vi "TI sbRIO Main (FPGA).vi"() -> ()   [LabVIEW 2019]
uses:
  Type Defs/Controller Names.ctl
  <vilib>/Platform/TimedLoop/XDataNode/timing_clust.ctl
  <vilib>/Platform/TimedLoop/XDataNode/nitl_modes.ctl
  <vilib>/Platform/TimedLoop/XDataNode/wakeup.ctl
  <vilib>/rvi/FXPMathLib/basic elements/FxpIntAccumulator/subVIs/nifxpmath_IntAccumulator_SimConfig.ctl
  <vilib>/rvi/FXPMathLib/FxpSqrt/subVIs/nifxpmath_Sqrt_SimConfig.ctl
  <vilib>/fxp/LVFixedPointOverflowPolicyTypeDef.ctl
  <vilib>/rvi/FXPMathLib/FxpDiv/subVIs/nifxpmath_Div_SimConfig.ctl
  <vilib>/rvi/Emulation/niFpgaGetClockAttributes.vi
  <vilib>/rvi/Emulation/niFpgaSctlEmulationGetInTimedLoop.vi
  <vilib>/rvi/Emulation/niFpgaEmulationReportErrorSimple.vi
  <vilib>/rvi/eio/common/nirviEmuTemplateMethod_errors.vi
  <vilib>/rvi/Emulation/niFpgaCriticalErrorInLSC.vi
  <vilib>/rvi/Analysis/common/codeGenErrors/XNode/niFpgaXNodeCodeGenErrorHandle.vi
  <vilib>/rvi/FXPMathLib/basic elements/FxpIntAccumulator/simVIs/DllFxpIntAccumulator_sub.vi
  <vilib>/rvi/FXPMathLib/FxpSqrt/simVIs/DllSqrtTemp_sub.vi
  <vilib>/rvi/Analysis/utilities/niFPGA Threshold Crossing Logic.vi
  <vilib>/rvi/FXPMathLib/FxpDiv/simVIs/DllFxpDivTemp_sub.vi
  <vilib>/eio/EIONode/EIONode.xnode
  <vilib>/rvi/Analysis/measure/butterworth/XNode/niFpgaButterworthFilter.xnode
  <vilib>/rvi/Analysis/measure/mean-var-std/XNode/niFpgaMean-Var-Std.xnode
  <vilib>/Platform/TimedLoop/XDataNode/XDataNode.xnode
  <vilib>/rvi/FXPMathLib/basic elements/FxpIntAccumulator/XNode/nifxpmath_IntAccumulator.xnode
  <vilib>/rvi/FXPMathLib/FxpMul/XNode/nifxpmath_Multiplier.xnode
  <vilib>/rvi/FXPMathLib/FxpAdd/XNode/nifxpmath_Add.xnode
  <vilib>/rvi/FXPMathLib/FxpSub/XNode/nifxpmath_Sub.xnode
  <vilib>/rvi/Analysis/measure/period/templates/niFPGA Period Edge Direction.ctl
  <vilib>/rvi/Analysis/measure/dc-rms/XNode/niFpgaDC-RMS.xnode
  <vilib>/rvi/FXPMathLib/FxpSqrt/XNode/nifxpmath_Sqrt.xnode
  <vilib>/rvi/Analysis/measure/period/XNode/niFpgaAnalogPeriod.xnode
  <vilib>/rvi/FXPMathLib/FxpDiv/XNode/nifxpmath_Div.xnode
  <vilib>/rvi/FXPMathLib/sim/FxpSim.dll
  <vilib>/Platform/TimedLoop/XDataNode/XDNodeRunTimeDep.lvlib
  <vilib>/rvi/DataTransferAndStorage/Container/XNode/niFpgaContainer.xnode
  <vilib>/rvi/FIFO/Fifo_Resource/niFpgaFifoEmulationRefIn.vi
panel:
  in  "DIO62":bool=TRUE
  in  "InvertPWM?":bool
  in  "PWM Duty":fxp<+,32,0>[](array[numeric])=[0.0, 0.0, 0.0, 0.0, 0.0, 0.0]
  in  "PWM Freq":fxp<+,32,0>=2.499902620911598e-06 caption="frequency (periods/tick)"
  in  "Enable Timers":bool[](array[boolean])=[FALSE, FALSE, FALSE, FALSE, FALSE, FALSE]
  in  "Controller Type:":T1
  in  "Conti Window":i32=434
  out "Temp 2":fxp<+/-,20,12> format="%#.1f"
  out "Currents (RMS)":fxp<+,26,7>[](array[numeric])
  out "Speed (RPM)":fxp<+,32,18>[](array[numeric])
  in  "Spike Window":i32=125
  in  "Min Window":i32=125
  in  "Max Window":i32=125
  in  "Disarm Level":i32=125
  in  "Arm Level":i32=125
  in  "PS Control":bool=TRUE
  out "Temp":fxp<+/-,20,12> format="%#.1f"
  in  "AO3":fxp<+/-,20,5>
  in  "AO2":fxp<+/-,20,5>
  in  "AO1":fxp<+/-,20,5>
  in  "AO0":fxp<+/-,20,5>
  in  "Kuhnke Window":i32=125
  in  "Speed Hysteresis":fxp<+,23,5>=1.0
  in  "Current Offset":fxp<+/-,18,7>=-60.09521484375 format="%#_14g"
  in  "Current Scale":fxp<+,16,5>=24.0380859375 format="%#_13g"
  out "Actual Loop Time":u32
  in  "Loop Timer (uSec)":u32=100
  in  "Current Offsets":fxp<+/-,24,7>[](array[numeric])=[0.0, 0.0, 0.0, 0.0, 0.0, 0.0]
  out "Elapsed Times":u64[](array[numeric])
  in  "Timer Resets":bool[](array[boolean])=[FALSE, FALSE, FALSE, FALSE, FALSE, FALSE]
  in  "Threshold":fxp<+/-,24,6>=1.0
  in  "Consec Samples":i32=125
  out "Actual Pump Starts":u32[](array[numeric])
  in  "Reset":bool
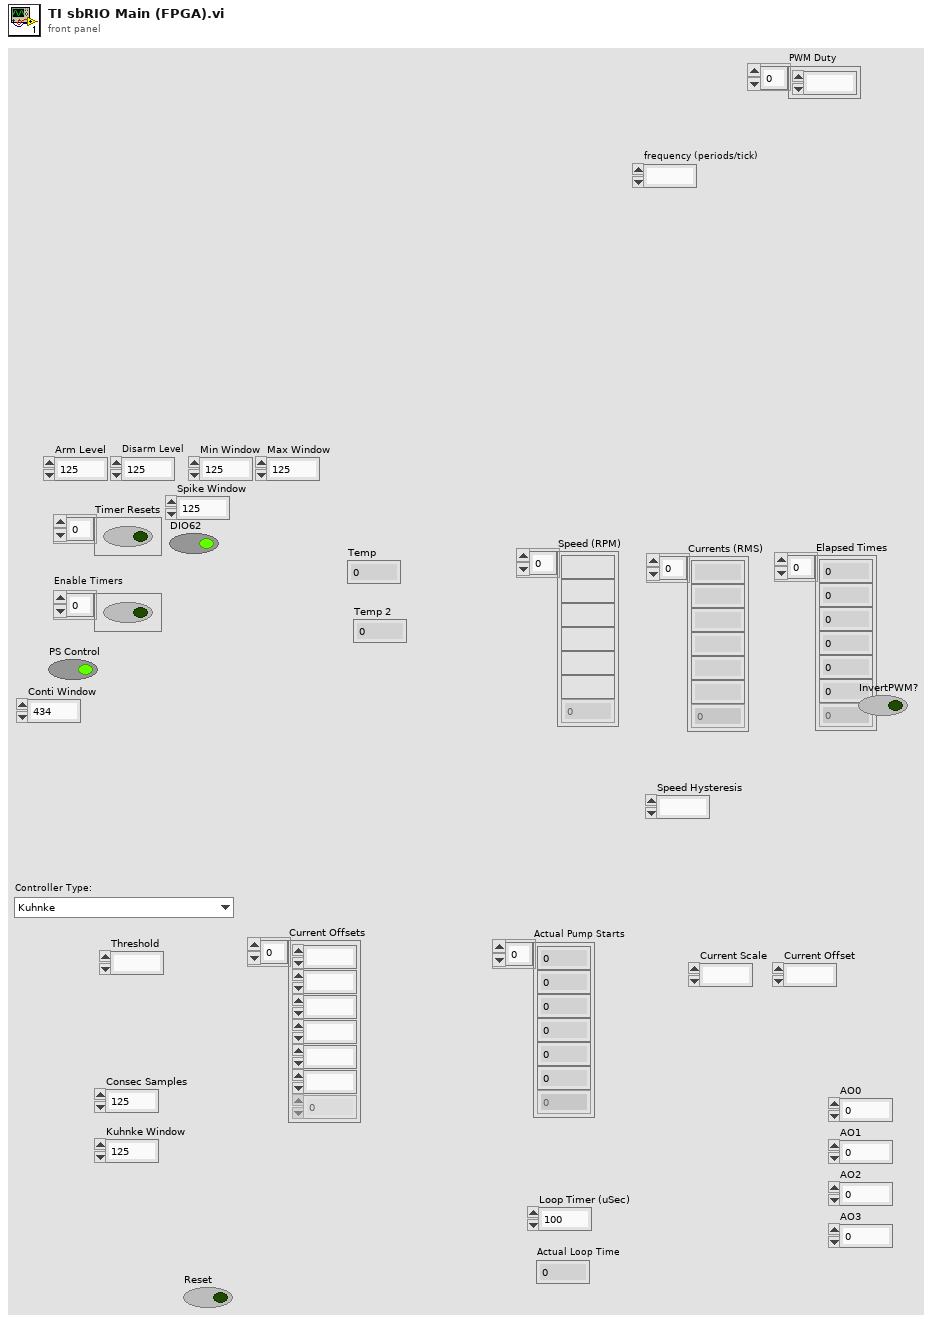
[diagram p1: front panel]
types:
  T1 = typedef "Controller Names.ctl" = enum16{"Kuhnke", "Conti", "Hella BLDC OL PWM", "Hella BLDC Turbine OL PWM", "Helbako", "TI PWM", "PSA", "Hella DC Gas", "Hella DC Diesel", "8 Comm", "10 Comm", "8 Comm Hella", "10 Comm Hella", "8 Comm Omron", "10 Comm Omron", "8 Comm Nissan", "10 Comm Nissan", "TI HP BLDC", "Mazda BLDC"}
  T2 = typedef "XDNodeRunTimeDep.lvlib/timing_clust.ctl" = cluster{"Expected End [f-1]":u64, "Actual End [f-1]":u64, "Finished Late? [f-1]":bool, "Expected End [i-1]":u64, "Actual End [i-1]":u64, "Finished Late? [i-1]":bool, "Expected Start [i]":u64, "Actual Start [i]":u64, "Expected Start [f]":u64, "Actual Start [f]":u64, "Source Name":string, "Structure Name":string, "Period":i64, "Deadline":i64, "Offset":i64, "Start":i64, "Priority":i32, "Timeout":i32, "Mode":T3, "Wakeup Reason":T4, "Error":errorcluster, "Source Type":string, "Secondary Source Type":string, "Global End Time":u64, "Global Start Time":u64, "Frame Duration":u64, "Iteration Duration":u64, "Assigned CPU":i32, "I/O Scan Engine Mode":u32}
  T3 = typedef "XDNodeRunTimeDep.lvlib/nitl_modes.ctl" = enum32{"No Change", "Process missed periods, maintain original phase", "Discard missed periods, maintain original phase", "Process missed periods, ignore original phase", "Discard missed periods, ignore original phase"}
  T4 = typedef "XDNodeRunTimeDep.lvlib/wakeup.ctl" = enum32{"Normal", "Aborted", "Asynchronous wakeup", "Timing source error", "Timed loop error", "Timeout"}
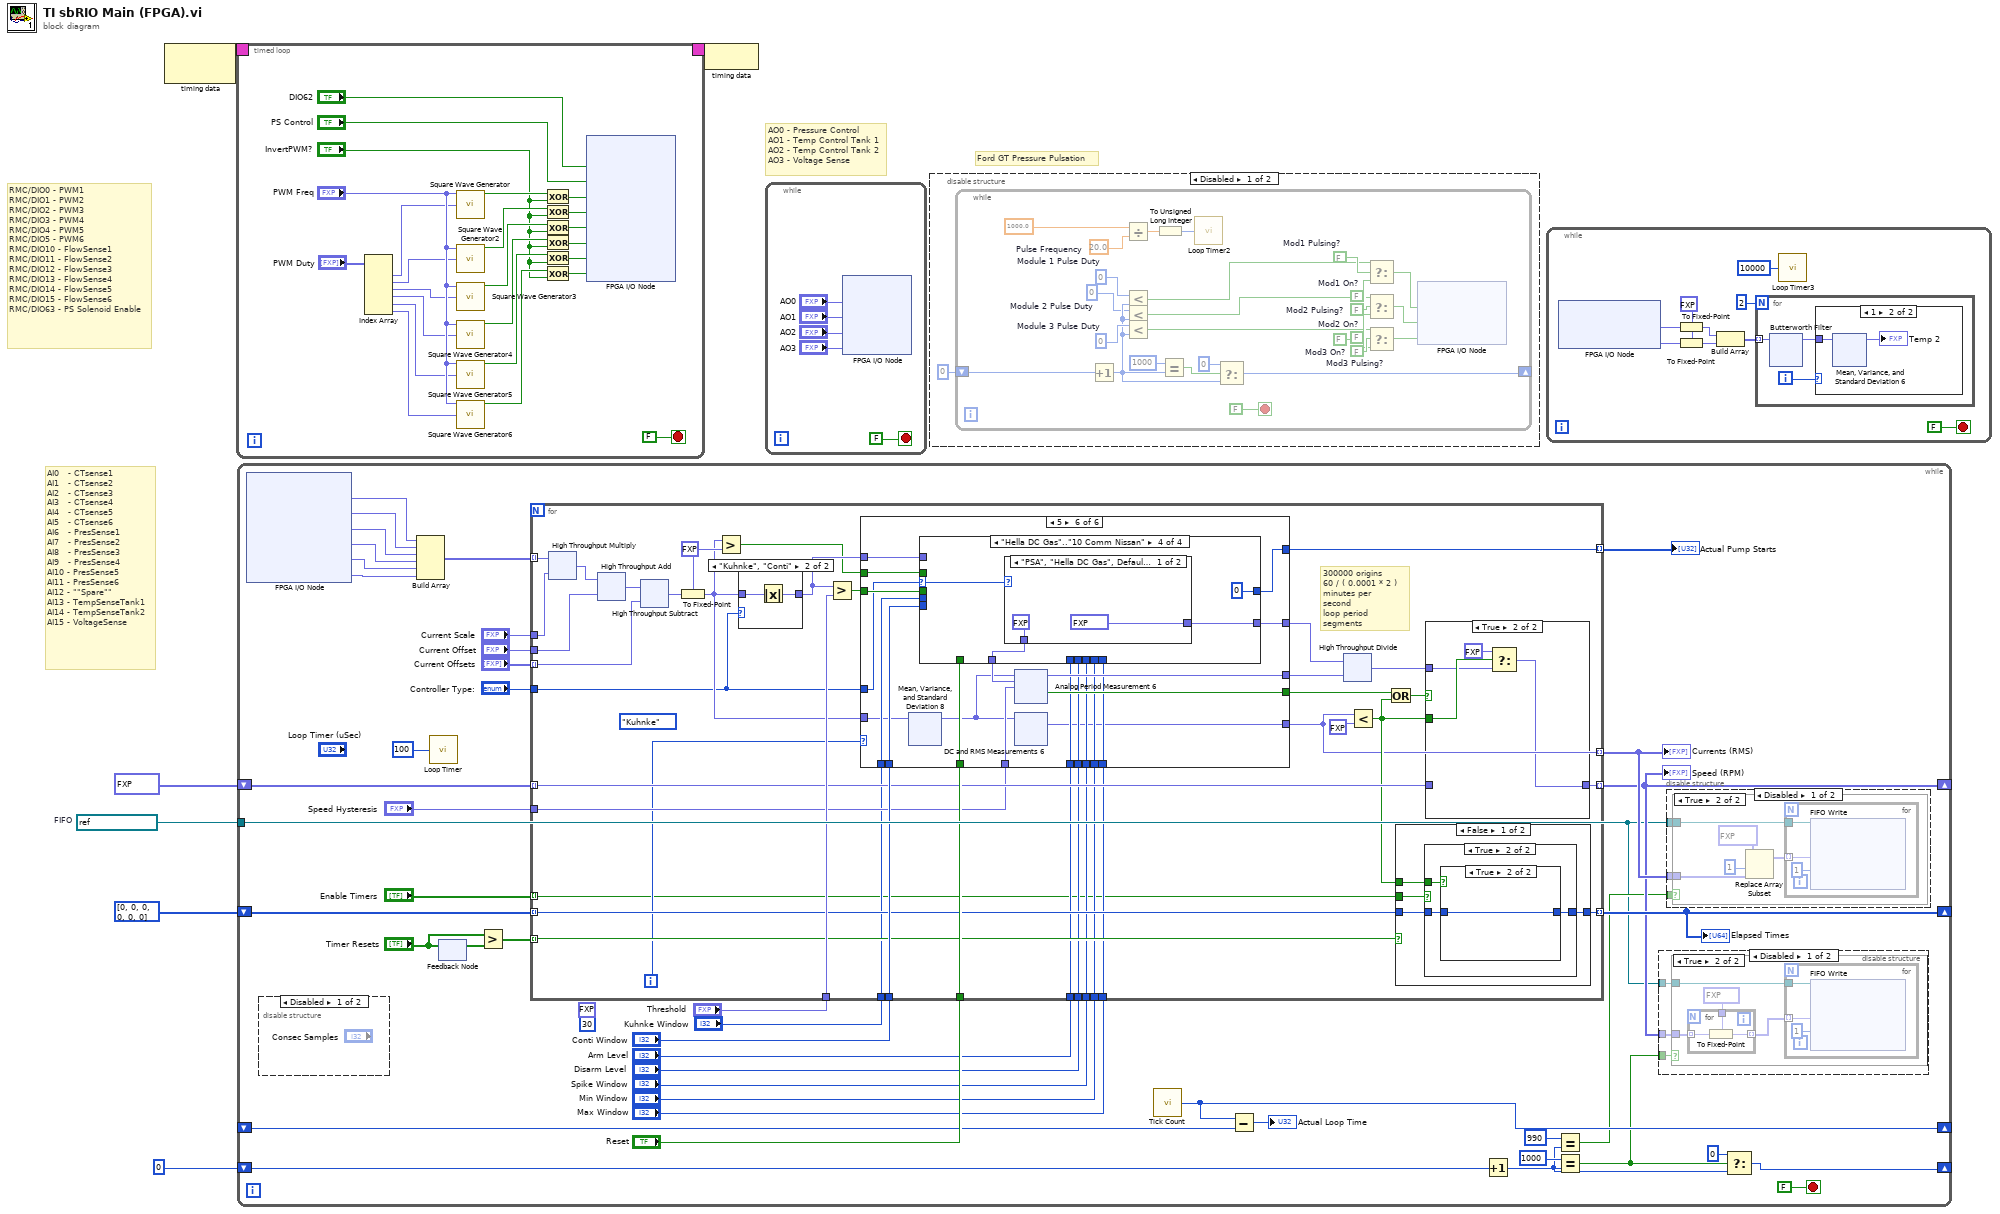
[diagram p0: block diagram]
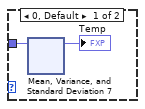
[diagram p3: hidden frame]
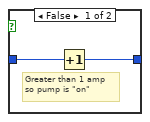
[diagram p11: hidden frame]
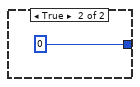
[diagram p12: hidden frame]
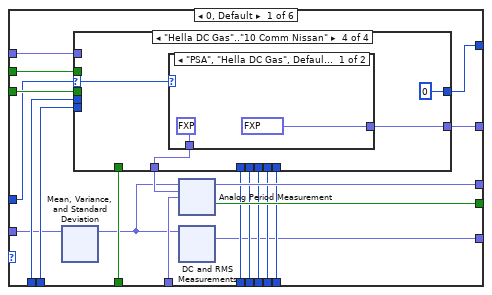
[diagram p14: hidden frame]
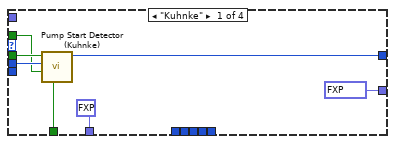
[diagram p15: hidden frame]
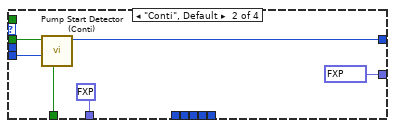
[diagram p16: hidden frame]
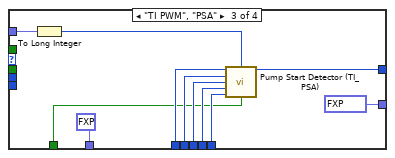
[diagram p17: hidden frame]
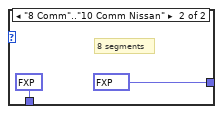
[diagram p18: hidden frame]
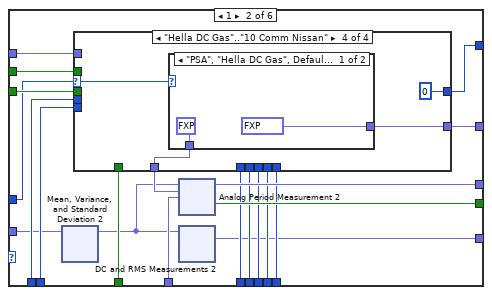
[diagram p19: hidden frame]
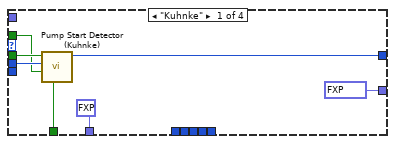
[diagram p20: hidden frame]
diagram:
  w3 = refnum<k21> "Current FIFO"  # FIFO
  # "Ford GT Pressure Pulsation"
  # "RMC/DIO0 - PWM1\nRMC/DIO1 - PWM2\nRMC/DIO2 - PWM3\nRMC/DIO3 - PWM4\nRMC/DIO4 - PWM5\nRMC/DIO5 - PWM6\nRMC/DIO10 - FlowSense1\nRMC/DIO11 - FlowSense2\nRMC/DIO12 - FlowSense3\nRMC/DIO13 - FlowSense4\nRMC/DIO14 - FlowSense5\nRMC/DIO15 - FlowSense6\nRMC/DIO63 - PS Solenoid Enable"
  # "AO0 - Pressure Control\nAO1 - Temp Control Tank 1\nAO2 - Temp Control Tank 2\nAO3 - Voltage Sense"
  # "AI0   - CTsense1\nAI1   - CTsense2\nAI2   - CTsense3\nAI3   - CTsense4\nAI4   - CTsense5\nAI5   - CTsense6\nAI6   - PresSense1\nAI7   - PresSense2\nAI8   - PresSense3\nAI9   - PresSense4\nAI10 - PresSense5\nAI11 - PresSense6\nAI12 - \"\"Spare\"\"\nAI13 - TempSenseTank1\nAI14 - TempSenseTank2\nAI15 - VoltageSense"
  n1 = node-c288() -> (w2:T2)  [unwired: 1 in]
  n2 = timed-loop {
    timing: w2 -> [_]
    timing-out: [_] -> w1
    stop <- FALSE stop-if-true
    n3 = Index Array(array="PWM Duty") -> (element #1=w14:fxp<+,32,0>, element #2=w13:fxp<+,32,0>, element #3=w12:fxp<+,32,0>, element #4=w11:fxp<+,32,0>, element #5=w10:fxp<+,32,0>, element #6=w9:fxp<+,32,0>)  [unwired: 6 in]
    n4 = call "Square Wave Generator"("frequency (periods/tick)"="PWM Freq", "duty cycle (periods)"=w14) -> ("square wave out"=w29:bool)  [unwired: 13 in]
    n5 = call "Square Wave Generator2"("frequency (periods/tick)"="PWM Freq", "duty cycle (periods)"=w13) -> ("square wave out"=w28:bool)  [unwired: 13 in]
    n6 = call "Square Wave Generator3"("frequency (periods/tick)"="PWM Freq", "duty cycle (periods)"=w12) -> ("square wave out"=w27:bool)  [unwired: 13 in]
    n7 = call "Square Wave Generator4"("frequency (periods/tick)"="PWM Freq", "duty cycle (periods)"=w11) -> ("square wave out"=w26:bool)  [unwired: 13 in]
    n8 = call "Square Wave Generator5"("frequency (periods/tick)"="PWM Freq", "duty cycle (periods)"=w10) -> ("square wave out"=w25:bool)  [unwired: 13 in]
    n9 = call "Square Wave Generator6"("frequency (periods/tick)"="PWM Freq", "duty cycle (periods)"=w9) -> ("square wave out"=w24:bool)  [unwired: 13 in]
    n10 = Exclusive Or(1:"InvertPWM?", 2:w29) -> (0:w22:bool)
    n11 = Exclusive Or(1:"InvertPWM?", 2:w28) -> (0:w21:bool)
    n12 = Exclusive Or(1:"InvertPWM?", 2:w27) -> (0:w20:bool)
    n13 = Exclusive Or(1:"InvertPWM?", 2:w26) -> (0:w19:bool)
    n14 = Exclusive Or(1:"InvertPWM?", 2:w25) -> (0:w18:bool)
    n15 = Exclusive Or(1:"InvertPWM?", 2:w24) -> (0:w17:bool)
    n16 = xnode "FPGA I/O Node"("RMC/DIO62"="DIO62", "RMC/DIO63"="PS Control", "RMC/DIO0"=w22, "RMC/DIO1"=w21, "RMC/DIO2"=w20, "RMC/DIO3"=w19, "RMC/DIO4"=w18, "RMC/DIO5"=w17) -> ()  [unwired: 9 in, 9 out]
  }
  n17 = while {
    shift-right: [w38] -> _
    shift-left: fxp<+,32,18>[] [0.0, 0.0, 0.0, 0.0, 0.0, 0.0] -> [w73]
    shift-right: [w71] -> _
    shift-left: u64[] [0, 0, 0, 0, 0, 0] -> [w72]
    shift-right: [w66] -> _
    shift-left: _ -> [w65]
    shift-right: [w42] -> _
    shift-left: u32 0 ("Tick Count(uSec)") -> [w45]
    tunnel: w3 -> [w35]
    stop <- FALSE stop-if-true
    (unwired) fxp<+/-,24,6> 1.0 ("Threshold")
    (unwired) 30 ("Kuhnke Window")
    n18 = xnode "FPGA I/O Node"() -> ("Current 1 (AI0)"=w56:fxp<+/-,24,5>, "Current 2 (AI1)"=w77:fxp<+/-,24,5>, "Current 3 (AI2)"=w60:fxp<+/-,24,5>, "Current 4 (AI3)"=w59:fxp<+/-,24,5>, "Current 5 (AI4)"=w58:fxp<+/-,24,5>, "Current 6 (AI5)"=w57:fxp<+/-,24,5>)  [unwired: 6 in, 6 out]
    n19 = disable-structure shown="Disabled" {
      frame Disabled {
      }
      frame Enabled {
      }
    }
    n20 = Build Array(w56, w77, w60, w59, w58, w57) -> (w74:fxp<+/-,24,5>[])
    n21 = call "Loop Timer"("Count(uSec)"=u32 100 ("Loop Timer (uSec)")) -> ()  [unwired: 1 out]
    n22 = feedback-in #1("Timer Resets") -> ()
    n23 = feedback #1() -> (w69:bool[])  [unwired: 1 in]
    n24 = Greater?(x="Timer Resets", y=w69) -> (0:w68:bool[])
    n25 = for {
      tunnel: "Conti Window" -> [w140]
      tunnel: [w139] -> w55 mode=indexing
      tunnel: "Threshold" -> [w138]
      tunnel: "Reset" -> [w136]
      tunnel: w74 -> [w120] mode=indexing
      tunnel: w72 -> [w127] mode=indexing
      tunnel: [w126] -> w71 mode=indexing
      tunnel: w73 -> [w131] mode=indexing
      tunnel: [w130] -> w38 mode=indexing
      tunnel: w68 -> [w125] mode=indexing
      tunnel: "Current Offsets" -> [w117] mode=indexing
      tunnel: [w105] -> w41 mode=indexing
      tunnel: "Current Scale" -> [w119]
      tunnel: "Current Offset" -> [w118]
      tunnel: "Speed Hysteresis" -> [w124]
      tunnel: "Kuhnke Window" -> [w123]
      tunnel: "Arm Level" -> [w114]
      tunnel: "Disarm Level" -> [w113]
      tunnel: "Spike Window" -> [w112]
      tunnel: "Min Window" -> [w111]
      tunnel: "Max Window" -> [w110]
      tunnel: "Controller Type:" -> [w103]
      tunnel: "Enable Timers" -> [w102] mode=indexing
      i -> [w106]
      (unwired) Controller_Names."Kuhnke" ("Controller Type:")
      w108 = fxp<+/-,26,7> 0.0 ("out")
      # "300000 origins\n60 / ( 0.0001 * 2 )\nminutes per second\nloop period\nsegments"
      n26 = xnode ("High Throughput Multiply")("x"=w120, "y"=w119) -> ("x*y"=w121:fxp<+/-,40,10>)
      n27 = xnode ("High Throughput Add")("x"=w121, "y"=w118) -> ("x+y"=w109:fxp<+/-,41,11>)
      n28 = xnode "High Throughput Subtract"("x"=w109, "y"=w117) -> ("x-y"=w122:fxp<+/-,42,12>)
      n29 = To Fixed-Point(fixed-point type=w108, number=w122) -> (fixed-point=w104:fxp<+/-,26,7>)
      n30 = Greater?(x=w104, y=w108) -> (0:w107:bool)
      n31 = case shown="\"Kuhnke\", \"Conti\"" w103 {
        tunnel: w104 -> [w141 w142]
        tunnel: [w141 w143] -> w116
        frame Default {
        }
        frame "Kuhnke", "Conti" {
          n32 = Absolute Value(x=w142) -> (abs(x)=w143:fxp<+,26,7>)
        }
      }
      n33 = Greater?(x=w116, y=w138) -> (0:w137:bool)
      n34 = case shown="5" w106 {
        tunnel: w137 -> [w208 w560 w912 w1264 w1616 w1968]
        tunnel: w140 -> [w207 w559 w911 w1263 w1615 w1967]
        tunnel: [w206 w558 w910 w1262 w1614 w1966] -> w139
        tunnel: w136 -> [w200 w552 w904 w1256 w1608 w1960]
        tunnel: w104 -> [w189 w541 w893 w1245 w1597 w1949]
        tunnel: [w191 w543 w895 w1247 w1599 w1951] -> w105
        tunnel: [w205 w557 w909 w1261 w1613 w1965] -> w132
        tunnel: [w204 w556 w908 w1260 w1612 w1964] -> w129
        tunnel: w103 -> [w203 w555 w907 w1259 w1611 w1963]
        tunnel: w124 -> [w202 w554 w906 w1258 w1610 w1962]
        tunnel: w123 -> [w201 w553 w905 w1257 w1609 w1961]
        tunnel: w116 -> [w199 w551 w903 w1255 w1607 w1959]
        tunnel: [w198 w550 w902 w1254 w1606 w1958] -> w115
        tunnel: w114 -> [w197 w549 w901 w1253 w1605 w1957]
        tunnel: w113 -> [w196 w548 w900 w1252 w1604 w1956]
        tunnel: w112 -> [w195 w547 w899 w1251 w1603 w1955]
        tunnel: w111 -> [w194 w546 w898 w1250 w1602 w1954]
        tunnel: w110 -> [w193 w545 w897 w1249 w1601 w1953]
        tunnel: w107 -> [w192 w544 w896 w1248 w1600 w1952]
        frame 0, Default {
          n35 = xnode ("Mean, Variance, and Standard Deviation")("input data"=w189) -> ("mean"=w188:fxp<+/-,26,7>)  [unwired: 1 in, 1 out]
          n36 = case shown="\"Hella DC Gas\"..\"10 Comm Nissan\"" w203 {
            selector: w203 -> [_ _ _ w311]
            tunnel: w208 -> [w290 w297 _ _]
            tunnel: w207 -> [_ w296 _ _]
            tunnel: [w289 w295 w301 u32 0 ("Restarts")] -> w206
            tunnel: w200 -> [w291 w294 w299 _]
            tunnel: w201 -> [w288 _ _ _]
            tunnel: w199 -> [_ _ w308 _]
            tunnel: [fxp<+,32,19> 300000.0 ("x") fxp<+,32,19> 300000.0 ("x") fxp<+,32,19> 300000.0 ("x") w310] -> w198
            tunnel: w197 -> [_ _ w306 _]
            tunnel: w196 -> [_ _ w305 _]
            tunnel: w195 -> [_ _ w304 _]
            tunnel: w194 -> [_ _ w303 _]
            tunnel: w193 -> [_ _ w302 _]
            tunnel: w192 -> [w286 _ _ _]
            tunnel: [fxp<+/-,24,7> 0.0 ("threshold level") fxp<+/-,24,7> 0.0 ("threshold level") fxp<+/-,24,7> 0.0 ("threshold level") w309] -> w190
            frame "Kuhnke" {
              n37 = call "Pump Start Detector (Kuhnke).vi"("Reset"=w291, "Pos?"=w286, "Window"=w288, "Pos Cross"=w290) -> ("Starts"=w289:u32)  [unwired: 6 in, 1 out]
            }
            frame "Conti", Default {
              n38 = call "Pump Start Detector (Conti).vi"("Reset"=w294, "Consec Samples"=w296, "Crossing?"=w297) -> ("Restarts"=w295:u32)  [unwired: 8 in]
            }
            frame "TI PWM", "PSA" {
              n39 = To Long Integer(number=w308) -> (32bit integer=w300:i32)
              n40 = call "Pump Start Detector (TI_PSA).vi"("Arm Level"=w306, "Level"=w300, "Disarm Level"=w305, "Spike Window"=w304, "Min Window"=w303, "Max Window"=w302, "Reset"=w299) -> ("Restarts"=w301:u32)  [unwired: 8 in]
            }
            frame "Hella DC Gas".."10 Comm Nissan" {
              n41 = case shown="\"PSA\", \"Hella DC Gas\", Default" w311 {
                tunnel: [fxp<+,32,19> 300000.0 ("x") fxp<+,32,19> 75000.0 ("x")] -> w310
                tunnel: [fxp<+/-,24,7> 0.0 ("threshold level") fxp<+/-,24,7> 6.75 ("threshold level")] -> w309
                frame "PSA", "Hella DC Gas", Default {
                }
                frame "8 Comm".."10 Comm Nissan" {
                  # "8 segments"
                }
              }
            }
          }
          n42 = xnode ("Analog Period Measurement")("input data"=w188, "threshold level"=w190, "hysteresis"=w202) -> ("period (samples)"=w204:fxp<+,32,16>, "output valid"=w205:bool)  [unwired: 2 in, 2 out]
          n43 = xnode ("DC and RMS Measurements")("input data"=w188) -> ("RMS"=w191:fxp<+,26,7>)  [unwired: 1 in, 1 out]
        }
        frame 1 {
          n44 = xnode ("Mean, Variance, and Standard Deviation 2")("input data"=w541) -> ("mean"=w540:fxp<+/-,26,7>)  [unwired: 1 in, 1 out]
          n45 = case shown="\"Hella DC Gas\"..\"10 Comm Nissan\"" w555 {
            selector: w555 -> [_ _ _ w663]
            tunnel: w560 -> [w642 w649 _ _]
            tunnel: w559 -> [_ w648 _ _]
            tunnel: [w641 w647 w653 u32 0 ("Restarts")] -> w558
            tunnel: w552 -> [w643 w646 w651 _]
            tunnel: w553 -> [w640 _ _ _]
            tunnel: w551 -> [_ _ w660 _]
            tunnel: [fxp<+,32,19> 300000.0 ("x") fxp<+,32,19> 300000.0 ("x") fxp<+,32,19> 300000.0 ("x") w662] -> w550
            tunnel: w549 -> [_ _ w658 _]
            tunnel: w548 -> [_ _ w657 _]
            tunnel: w547 -> [_ _ w656 _]
            tunnel: w546 -> [_ _ w655 _]
            tunnel: w545 -> [_ _ w654 _]
            tunnel: w544 -> [w638 _ _ _]
            tunnel: [fxp<+/-,24,7> 0.0 ("threshold level") fxp<+/-,24,7> 0.0 ("threshold level") fxp<+/-,24,7> 0.0 ("threshold level") w661] -> w542
            frame "Kuhnke" {
              n46 = call "Pump Start Detector (Kuhnke).vi"("Reset"=w643, "Pos?"=w638, "Window"=w640, "Pos Cross"=w642) -> ("Starts"=w641:u32)  [unwired: 6 in, 1 out]
            }
            frame "Conti", Default {
              n47 = call "Pump Start Detector (Conti).vi"("Reset"=w646, "Consec Samples"=w648, "Crossing?"=w649) -> ("Restarts"=w647:u32)  [unwired: 8 in]
            }
            frame "TI PWM", "PSA" {
              n48 = To Long Integer(number=w660) -> (32bit integer=w652:i32)
              n49 = call "Pump Start Detector (TI_PSA).vi"("Arm Level"=w658, "Level"=w652, "Disarm Level"=w657, "Spike Window"=w656, "Min Window"=w655, "Max Window"=w654, "Reset"=w651) -> ("Restarts"=w653:u32)  [unwired: 8 in]
            }
            frame "Hella DC Gas".."10 Comm Nissan" {
              n50 = case shown="\"PSA\", \"Hella DC Gas\", Default" w663 {
                tunnel: [fxp<+,32,19> 300000.0 ("x") fxp<+,32,19> 75000.0 ("x")] -> w662
                tunnel: [fxp<+/-,24,7> 0.0 ("threshold level") fxp<+/-,24,7> 6.75 ("threshold level")] -> w661
                frame "PSA", "Hella DC Gas", Default {
                }
                frame "8 Comm".."10 Comm Nissan" {
                  # "8 segments"
                }
              }
            }
          }
          n51 = xnode ("Analog Period Measurement 2")("input data"=w540, "threshold level"=w542, "hysteresis"=w554) -> ("period (samples)"=w556:fxp<+,32,16>, "output valid"=w557:bool)  [unwired: 2 in, 2 out]
          n52 = xnode ("DC and RMS Measurements 2")("input data"=w540) -> ("RMS"=w543:fxp<+,26,7>)  [unwired: 1 in, 1 out]
        }
        frame 2 {
          n53 = xnode ("Mean, Variance, and Standard Deviation 3")("input data"=w893) -> ("mean"=w892:fxp<+/-,26,7>)  [unwired: 1 in, 1 out]
          n54 = case shown="\"Hella DC Gas\"..\"10 Comm Nissan\"" w907 {
            selector: w907 -> [_ _ _ w1015]
            tunnel: w912 -> [w994 w1001 _ _]
            tunnel: w911 -> [_ w1000 _ _]
            tunnel: [w993 w999 w1005 u32 0 ("Restarts")] -> w910
            tunnel: w904 -> [w995 w998 w1003 _]
            tunnel: w905 -> [w992 _ _ _]
            tunnel: w903 -> [_ _ w1012 _]
            tunnel: [fxp<+,32,19> 300000.0 ("x") fxp<+,32,19> 300000.0 ("x") fxp<+,32,19> 300000.0 ("x") w1014] -> w902
            tunnel: w901 -> [_ _ w1010 _]
            tunnel: w900 -> [_ _ w1009 _]
            tunnel: w899 -> [_ _ w1008 _]
            tunnel: w898 -> [_ _ w1007 _]
            tunnel: w897 -> [_ _ w1006 _]
            tunnel: w896 -> [w990 _ _ _]
            tunnel: [fxp<+/-,24,7> 0.0 ("threshold level") fxp<+/-,24,7> 0.0 ("threshold level") fxp<+/-,24,7> 0.0 ("threshold level") w1013] -> w894
            frame "Kuhnke" {
              n55 = call "Pump Start Detector (Kuhnke).vi"("Reset"=w995, "Pos?"=w990, "Window"=w992, "Pos Cross"=w994) -> ("Starts"=w993:u32)  [unwired: 6 in, 1 out]
            }
            frame "Conti", Default {
              n56 = call "Pump Start Detector (Conti).vi"("Reset"=w998, "Consec Samples"=w1000, "Crossing?"=w1001) -> ("Restarts"=w999:u32)  [unwired: 8 in]
            }
            frame "TI PWM", "PSA" {
              n57 = To Long Integer(number=w1012) -> (32bit integer=w1004:i32)
              n58 = call "Pump Start Detector (TI_PSA).vi"("Arm Level"=w1010, "Level"=w1004, "Disarm Level"=w1009, "Spike Window"=w1008, "Min Window"=w1007, "Max Window"=w1006, "Reset"=w1003) -> ("Restarts"=w1005:u32)  [unwired: 8 in]
            }
            frame "Hella DC Gas".."10 Comm Nissan" {
              n59 = case shown="\"PSA\", \"Hella DC Gas\", Default" w1015 {
                tunnel: [fxp<+,32,19> 300000.0 ("x") fxp<+,32,19> 75000.0 ("x")] -> w1014
                tunnel: [fxp<+/-,24,7> 0.0 ("threshold level") fxp<+/-,24,7> 6.75 ("threshold level")] -> w1013
                frame "PSA", "Hella DC Gas", Default {
                }
                frame "8 Comm".."10 Comm Nissan" {
                  # "8 segments"
                }
              }
            }
          }
          n60 = xnode ("Analog Period Measurement 3")("input data"=w892, "threshold level"=w894, "hysteresis"=w906) -> ("period (samples)"=w908:fxp<+,32,16>, "output valid"=w909:bool)  [unwired: 2 in, 2 out]
          n61 = xnode ("DC and RMS Measurements 3")("input data"=w892) -> ("RMS"=w895:fxp<+,26,7>)  [unwired: 1 in, 1 out]
        }
        frame 3 {
          n62 = xnode ("Mean, Variance, and Standard Deviation 4")("input data"=w1245) -> ("mean"=w1244:fxp<+/-,26,7>)  [unwired: 1 in, 1 out]
          n63 = case shown="\"Hella DC Gas\"..\"10 Comm Nissan\"" w1259 {
            selector: w1259 -> [_ _ _ w1367]
            tunnel: w1264 -> [w1346 w1353 _ _]
            tunnel: w1263 -> [_ w1352 _ _]
            tunnel: [w1345 w1351 w1357 u32 0 ("Restarts")] -> w1262
            tunnel: w1256 -> [w1347 w1350 w1355 _]
            tunnel: w1257 -> [w1344 _ _ _]
            tunnel: w1255 -> [_ _ w1364 _]
            tunnel: [fxp<+,32,19> 300000.0 ("x") fxp<+,32,19> 300000.0 ("x") fxp<+,32,19> 300000.0 ("x") w1366] -> w1254
            tunnel: w1253 -> [_ _ w1362 _]
            tunnel: w1252 -> [_ _ w1361 _]
            tunnel: w1251 -> [_ _ w1360 _]
            tunnel: w1250 -> [_ _ w1359 _]
            tunnel: w1249 -> [_ _ w1358 _]
            tunnel: w1248 -> [w1342 _ _ _]
            tunnel: [fxp<+/-,24,7> 0.0 ("threshold level") fxp<+/-,24,7> 0.0 ("threshold level") fxp<+/-,24,7> 0.0 ("threshold level") w1365] -> w1246
            frame "Kuhnke" {
              n64 = call "Pump Start Detector (Kuhnke).vi"("Reset"=w1347, "Pos?"=w1342, "Window"=w1344, "Pos Cross"=w1346) -> ("Starts"=w1345:u32)  [unwired: 6 in, 1 out]
            }
            frame "Conti", Default {
              n65 = call "Pump Start Detector (Conti).vi"("Reset"=w1350, "Consec Samples"=w1352, "Crossing?"=w1353) -> ("Restarts"=w1351:u32)  [unwired: 8 in]
            }
            frame "TI PWM", "PSA" {
              n66 = To Long Integer(number=w1364) -> (32bit integer=w1356:i32)
              n67 = call "Pump Start Detector (TI_PSA).vi"("Arm Level"=w1362, "Level"=w1356, "Disarm Level"=w1361, "Spike Window"=w1360, "Min Window"=w1359, "Max Window"=w1358, "Reset"=w1355) -> ("Restarts"=w1357:u32)  [unwired: 8 in]
            }
            frame "Hella DC Gas".."10 Comm Nissan" {
              n68 = case shown="\"PSA\", \"Hella DC Gas\", Default" w1367 {
                tunnel: [fxp<+,32,19> 300000.0 ("x") fxp<+,32,19> 75000.0 ("x")] -> w1366
                tunnel: [fxp<+/-,24,7> 0.0 ("threshold level") fxp<+/-,24,7> 6.75 ("threshold level")] -> w1365
                frame "PSA", "Hella DC Gas", Default {
                }
                frame "8 Comm".."10 Comm Nissan" {
                  # "8 segments"
                }
              }
            }
          }
          n69 = xnode ("Analog Period Measurement 4")("input data"=w1244, "threshold level"=w1246, "hysteresis"=w1258) -> ("period (samples)"=w1260:fxp<+,32,16>, "output valid"=w1261:bool)  [unwired: 2 in, 2 out]
          n70 = xnode ("DC and RMS Measurements 4")("input data"=w1244) -> ("RMS"=w1247:fxp<+,26,7>)  [unwired: 1 in, 1 out]
        }
        frame 4 {
          n71 = xnode ("Mean, Variance, and Standard Deviation 5")("input data"=w1597) -> ("mean"=w1596:fxp<+/-,26,7>)  [unwired: 1 in, 1 out]
          n72 = case shown="\"Hella DC Gas\"..\"10 Comm Nissan\"" w1611 {
            selector: w1611 -> [_ _ _ w1719]
            tunnel: w1616 -> [w1698 w1705 _ _]
            tunnel: w1615 -> [_ w1704 _ _]
            tunnel: [w1697 w1703 w1709 u32 0 ("Restarts")] -> w1614
            tunnel: w1608 -> [w1699 w1702 w1707 _]
            tunnel: w1609 -> [w1696 _ _ _]
            tunnel: w1607 -> [_ _ w1716 _]
            tunnel: [fxp<+,32,19> 300000.0 ("x") fxp<+,32,19> 300000.0 ("x") fxp<+,32,19> 300000.0 ("x") w1718] -> w1606
            tunnel: w1605 -> [_ _ w1714 _]
            tunnel: w1604 -> [_ _ w1713 _]
            tunnel: w1603 -> [_ _ w1712 _]
            tunnel: w1602 -> [_ _ w1711 _]
            tunnel: w1601 -> [_ _ w1710 _]
            tunnel: w1600 -> [w1694 _ _ _]
            tunnel: [fxp<+/-,24,7> 0.0 ("threshold level") fxp<+/-,24,7> 0.0 ("threshold level") fxp<+/-,24,7> 0.0 ("threshold level") w1717] -> w1598
            frame "Kuhnke" {
              n73 = call "Pump Start Detector (Kuhnke).vi"("Reset"=w1699, "Pos?"=w1694, "Window"=w1696, "Pos Cross"=w1698) -> ("Starts"=w1697:u32)  [unwired: 6 in, 1 out]
            }
            frame "Conti", Default {
              n74 = call "Pump Start Detector (Conti).vi"("Reset"=w1702, "Consec Samples"=w1704, "Crossing?"=w1705) -> ("Restarts"=w1703:u32)  [unwired: 8 in]
            }
            frame "TI PWM", "PSA" {
              n75 = To Long Integer(number=w1716) -> (32bit integer=w1708:i32)
              n76 = call "Pump Start Detector (TI_PSA).vi"("Arm Level"=w1714, "Level"=w1708, "Disarm Level"=w1713, "Spike Window"=w1712, "Min Window"=w1711, "Max Window"=w1710, "Reset"=w1707) -> ("Restarts"=w1709:u32)  [unwired: 8 in]
            }
            frame "Hella DC Gas".."10 Comm Nissan" {
              n77 = case shown="\"PSA\", \"Hella DC Gas\", Default" w1719 {
                tunnel: [fxp<+,32,19> 300000.0 ("x") fxp<+,32,19> 75000.0 ("x")] -> w1718
                tunnel: [fxp<+/-,24,7> 0.0 ("threshold level") fxp<+/-,24,7> 6.75 ("threshold level")] -> w1717
                frame "PSA", "Hella DC Gas", Default {
                }
                frame "8 Comm".."10 Comm Nissan" {
                  # "8 segments"
                }
              }
            }
          }
          n78 = xnode ("Analog Period Measurement 5")("input data"=w1596, "threshold level"=w1598, "hysteresis"=w1610) -> ("period (samples)"=w1612:fxp<+,32,16>, "output valid"=w1613:bool)  [unwired: 2 in, 2 out]
          n79 = xnode ("DC and RMS Measurements 5")("input data"=w1596) -> ("RMS"=w1599:fxp<+,26,7>)  [unwired: 1 in, 1 out]
        }
        frame 5 {
          n80 = xnode ("Mean, Variance, and Standard Deviation 8")("input data"=w1949) -> ("mean"=w1948:fxp<+/-,26,7>)  [unwired: 1 in, 1 out]
          n81 = case shown="\"Hella DC Gas\"..\"10 Comm Nissan\"" w1963 {
            selector: w1963 -> [_ _ _ w2071]
            tunnel: w1968 -> [w2050 w2057 _ _]
            tunnel: w1967 -> [_ w2056 _ _]
            tunnel: [w2049 w2055 w2061 u32 0 ("Restarts")] -> w1966
            tunnel: w1960 -> [w2051 w2054 w2059 _]
            tunnel: w1961 -> [w2048 _ _ _]
            tunnel: w1959 -> [_ _ w2068 _]
            tunnel: [fxp<+,32,19> 300000.0 ("x") fxp<+,32,19> 300000.0 ("x") fxp<+,32,19> 300000.0 ("x") w2070] -> w1958
            tunnel: w1957 -> [_ _ w2066 _]
            tunnel: w1956 -> [_ _ w2065 _]
            tunnel: w1955 -> [_ _ w2064 _]
            tunnel: w1954 -> [_ _ w2063 _]
            tunnel: w1953 -> [_ _ w2062 _]
            tunnel: w1952 -> [w2046 _ _ _]
            tunnel: [fxp<+/-,24,7> 0.0 ("threshold level") fxp<+/-,24,7> 0.0 ("threshold level") fxp<+/-,24,7> 0.0 ("threshold level") w2069] -> w1950
            frame "Kuhnke" {
              n82 = call "Pump Start Detector (Kuhnke).vi"("Reset"=w2051, "Pos?"=w2046, "Window"=w2048, "Pos Cross"=w2050) -> ("Starts"=w2049:u32)  [unwired: 6 in, 1 out]
            }
            frame "Conti", Default {
              n83 = call "Pump Start Detector (Conti).vi"("Reset"=w2054, "Consec Samples"=w2056, "Crossing?"=w2057) -> ("Restarts"=w2055:u32)  [unwired: 8 in]
            }
            frame "TI PWM", "PSA" {
              n84 = To Long Integer(number=w2068) -> (32bit integer=w2060:i32)
              n85 = call "Pump Start Detector (TI_PSA).vi"("Arm Level"=w2066, "Level"=w2060, "Disarm Level"=w2065, "Spike Window"=w2064, "Min Window"=w2063, "Max Window"=w2062, "Reset"=w2059) -> ("Restarts"=w2061:u32)  [unwired: 8 in]
            }
            frame "Hella DC Gas".."10 Comm Nissan" {
              n86 = case shown="\"PSA\", \"Hella DC Gas\", Default" w2071 {
                tunnel: [fxp<+,32,19> 300000.0 ("x") fxp<+,32,19> 75000.0 ("x")] -> w2070
                tunnel: [fxp<+/-,24,7> 0.0 ("threshold level") fxp<+/-,24,7> 6.75 ("threshold level")] -> w2069
                frame "PSA", "Hella DC Gas", Default {
                }
                frame "8 Comm".."10 Comm Nissan" {
                  # "8 segments"
                }
              }
            }
          }
          n87 = xnode ("Analog Period Measurement 6")("input data"=w1948, "threshold level"=w1950, "hysteresis"=w1962) -> ("period (samples)"=w1964:fxp<+,32,16>, "output valid"=w1965:bool)  [unwired: 2 in, 2 out]
          n88 = xnode ("DC and RMS Measurements 6")("input data"=w1948) -> ("RMS"=w1951:fxp<+,26,7>)  [unwired: 1 in, 1 out]
        }
      }
      n89 = xnode "High Throughput Divide"("x"=w115, "y"=w129) -> ("x/y"=w133:fxp<+,32,18>)
      n90 = Less?(x=w105, y=fxp<+,24,6> 1.0 ("current threshold")) -> (x < y?=w128:bool)
      n91 = Or(x=w132, y=w128) -> (x .or. y?=w134:bool)
      n92 = case shown="False" w125 {
        tunnel: w128 -> [w147 _]
        tunnel: w127 -> [w146 _]
        tunnel: [w145 u64 0] -> w126
        tunnel: w102 -> [w144 _]
        frame False {
          n93 = case shown="True" w144 {
            tunnel: w147 -> [_ w151]
            tunnel: w146 -> [w148 w150]
            tunnel: [w148 w149] -> w145
            frame False {
            }
            frame True {
              n94 = case shown="True" w151 {
                tunnel: w150 -> [w153 w154]
                tunnel: [w152 w154] -> w149
                frame False {
                  # "Greater than 1 amp\nso pump is \"on\""
                  n95 = Increment(x=w153) -> (x+1=w152:u64)
                }
                frame True {
                }
              }
            }
          }
        }
        frame True {
        }
      }
      n96 = case shown="True" w134 {
        tunnel: w133 -> [_ w158]
        tunnel: w128 -> [_ w159]
        tunnel: w131 -> [w156 _]
        tunnel: [w156 w157] -> w130
        frame False {
        }
        frame True {
          n97 = Select(t=fxp<+,32,18> 0.0 ("input data"), s=w159, f=w158) -> (s? t:f=w157:fxp<+,32,18>)
        }
      }
    }
    "Actual Pump Starts" <- w55
    "Elapsed Times" <- w71
    "Speed (RPM)" <- w38
    "Currents (RMS)" <- w41
    n98 = call "Tick Count"() -> ("Tick Count(uSec)"=w66:u32)
    n99 = Subtract(x=w66, y=w65) -> (x-y=→"Actual Loop Time":u32)
    n100 = Increment(x=w45) -> (x+1=w40:u32)
    n101 = Equal?(x=u32 990, y=w40) -> (x = y?=w37:bool)
    n102 = Equal?(x=u32 1000, y=w40) -> (x = y?=w36:bool)
    n103 = disable-structure shown="Disabled" {
      disable-tunnel: w38 -> [w91 _]
      disable-tunnel: w36 -> [w90 _]
      disable-tunnel: w35 -> [w89 _]
      frame Disabled {
        n104 = case shown="True" w90 {
          tunnel: w89 -> [_ w95]
          tunnel: w91 -> [_ w93]
          frame False {
          }
          frame True {
            n105 = for {
              tunnel: fxp<+/-,35,16> -32768.0 ("Element") -> [w98]
              tunnel: w93 -> [w97] mode=indexing
              tunnel: [w96] -> w92 mode=indexing
              n106 = To Fixed-Point(fixed-point type=w98, number=w97) -> (fixed-point=w96:fxp<+/-,35,16>)
            }
            n107 = for {
              tunnel: w95 -> [w101]
              tunnel: w92 -> [w99] mode=indexing
              n108 = xnode ("FIFO Write")("Element"=w99, "Timeout"=1, "FIFO In"=w101) -> ()  [unwired: 2 out]
            }
          }
        }
      }
      frame Enabled {
      }
    }
    n109 = disable-structure shown="Disabled" {
      disable-tunnel: w41 -> [w80 _]
      disable-tunnel: w37 -> [w79 _]
      disable-tunnel: w35 -> [w78 _]
      frame Disabled {
        n110 = case shown="True" w79 {
          tunnel: w78 -> [_ w85]
          tunnel: w80 -> [_ w84]
          frame False {
          }
          frame True {
            n111 = Replace Array Subset(array=fxp<+/-,35,16>[] [-32768.0, -32768.0, -32768.0, -32768.0, -32768.0, -32768.0, -32768.0], new element=w84, index=1) -> (w82:fxp<+/-,35,16>[])
            n112 = for {
              tunnel: w85 -> [w88]
              tunnel: w82 -> [w86] mode=indexing
              n113 = xnode ("FIFO Write")("Element"=w86, "Timeout"=1, "FIFO In"=w88) -> ()  [unwired: 2 out]
            }
          }
        }
      }
      frame Enabled {
      }
    }
    n114 = Select(t=u32 0 ("x"), s=w36, f=w40) -> (s? t:f=w42:u32)
  }
  n115 = node-c288(w1) -> ()
  n116 = while {
    stop <- FALSE stop-if-true
    n117 = xnode "FPGA I/O Node"("AO0"="AO0", "AO1"="AO1", "AO2"="AO2", "AO3"="AO3") -> ()  [unwired: 4 in, 4 out]
  }
  n118 = disable-structure shown="Disabled" {
    frame Disabled {
      n119 = while {
        shift-right: [w2321] -> _
        shift-left: i16 0 -> [w2326]
        stop <- FALSE stop-if-true
        w2312 = FALSE  # Mod3 On?
        w2313 = FALSE  # Mod3 Pulsing?
        w2315 = FALSE  # Mod2 On?
        w2314 = FALSE  # Mod2 Pulsing?
        w2316 = FALSE  # Mod1 On?
        w2317 = FALSE  # Mod1 Pulsing?
        w2322 = i16 0  # Module 3 Pulse Duty
        w2318 = i16 0  # Module 2 Pulse Duty
        w2319 = i16 0  # Module 1 Pulse Duty
        w2329 = sgl 20.0  # Pulse Frequency
        n120 = Increment(x=w2326) -> (x+1=w2320:i16)
        n121 = Divide(x=sgl 1000.0, y=w2329) -> (x/y=w2328:sgl)
        n122 = Less?(x=w2319, y=w2320) -> (x < y?=w2309:bool)
        n123 = Less?(x=w2318, y=w2320) -> (x < y?=w2310:bool)
        n124 = Less?(x=w2322, y=w2320) -> (x < y?=w2311:bool)
        n125 = To Unsigned Long Integer(number=w2328) -> (unsigned 32bit integer=w2327:u32)
        n126 = Equal?(x=i16 1000, y=w2320) -> (x = y?=w2324:bool)
        n127 = call "Loop Timer2"("Count(uSec)"=w2327) -> ()  [unwired: 1 out]
        n128 = Select(t=i16 0, s=w2324, f=w2320) -> (s? t:f=w2321:i16)
        n129 = Select(t=w2309, s=w2317, f=w2316) -> (s? t:f=w2306:bool)
        n130 = Select(t=w2310, s=w2314, f=w2315) -> (s? t:f=w2307:bool)
        n131 = Select(t=w2311, s=w2313, f=w2312) -> (s? t:f=w2308:bool)
        n132 = xnode "FPGA I/O Node"("RMC/DIO15"=w2306, "RMC/DIO31"=w2307, "RMC/DIO47"=w2308) -> ()  [unwired: 3 in, 3 out]
      }
    }
    frame Enabled {
    }
  }
  n133 = while {
    stop <- FALSE stop-if-true
    w2334 = fxp<+/-,16,8> 0.0
    n134 = xnode "FPGA I/O Node"() -> ("Temp 1 (AI13)"=w2338:fxp<+/-,24,5>, "Temp 2 (AI14)"=w2336:fxp<+/-,24,5>)  [unwired: 2 in, 2 out]
    n135 = To Fixed-Point(fixed-point type=w2334, number=w2338) -> (fixed-point=w2337:fxp<+/-,16,8>)
    n136 = To Fixed-Point(fixed-point type=w2334, number=w2336) -> (fixed-point=w2335:fxp<+/-,16,8>)
    n137 = Build Array(w2337, w2335) -> (w2333:fxp<+/-,16,8>[])
    n138 = for {
      N: 2 -> [_]
      tunnel: w2333 -> [w2343] mode=indexing
      i -> [w2342]
      n139 = xnode "Butterworth Filter"("input data"=w2343) -> ("output data"=w2341:fxp<+/-,20,12>)  [unwired: 2 in, 1 out]
      n140 = case shown="1" w2342 {
        tunnel: w2341 -> [w2344 w2422]
        frame 0, Default {
          n141 = xnode ("Mean, Variance, and Standard Deviation 7")("input data"=w2344) -> ("mean"=→"Temp":fxp<+/-,20,12>)  [unwired: 1 in, 1 out]
        }
        frame 1 {
          n142 = xnode ("Mean, Variance, and Standard Deviation 6")("input data"=w2422) -> ("mean"=→"Temp 2":fxp<+/-,20,12>)  [unwired: 1 in, 1 out]
        }
      }
    }
    n143 = call "Loop Timer3"("Count(uSec)"=u32 10000) -> ()  [unwired: 1 out]
  }
